vi "Main panel.vi"() -> ()   [LabVIEW 2019]
uses:
  <vilib>/Platform/TimedLoop/XDataNode/timing_clust.ctl
  <vilib>/Platform/TimedLoop/XDataNode/nitl_modes.ctl
  <vilib>/Platform/TimedLoop/XDataNode/wakeup.ctl
  <vilib>/myRIO/Instrument Drivers/Onboard IO/AI/typedefs/AI Reference.ctl
  <vilib>/myRIO/Common/Instrument Driver Framework/Utilities/typedefs/myRIO Generic Hardware Reference.ctl
  <vilib>/myRIO/Common/Instrument Driver Framework/Utilities/typedefs/Hardware Version Enum.ctl
  <vilib>/myRIO/Common/Instrument Driver Framework/Utilities/typedefs/myRIO v1.0 Reference.ctl
  <vilib>/myRIO/Common/Instrument Driver Framework/Utilities/typedefs/Generic FPGA Reference.ctl
  <vilib>/myRIO/Common/Instrument Driver Framework/myRIO v1.0/AI/typedefs/AI Channels List.ctl
  <vilib>/myRIO/Common/Instrument Driver Framework/myRIO v1.0/AI/typedefs/AI Channels Enum.ctl
  <vilib>/myRIO/Common/Instrument Driver Framework/Utilities/typedefs/Analog Scaling Constants List.ctl
  <vilib>/myRIO/Common/Instrument Driver Framework/Utilities/typedefs/Analog Scaling Constants.ctl
  <vilib>/userdefined/High Color/nirio_resource_hc.ctl
  <vilib>/myRIO/Instrument Drivers/Onboard IO/AO/typedefs/AO Reference.ctl
  <vilib>/myRIO/Common/Instrument Driver Framework/myRIO v1.0/AO/typedefs/AO Channels List.ctl
  <vilib>/myRIO/Common/Instrument Driver Framework/myRIO v1.0/AO/typedefs/AO Channels Enum.ctl
  <vilib>/myRIO/Common/Instrument Driver Framework/Utilities/vis/Is FPGA Ref Available.vi
  <vilib>/myRIO/Common/Instrument Driver Framework/myRIO v1.0/AI/vis/myRIO v1.1 Open AI.vi
  <vilib>/myRIO/Instrument Drivers/Onboard IO/AI/vis/Read.vi
  <vilib>/myRIO/Common/Instrument Driver Framework/myRIO v1.0/AO/vis/myRIO v1.1 Open AO.vi
  <vilib>/myRIO/Instrument Drivers/Onboard IO/AO/vis/Write.vi
  <vilib>/myRIO/Common/Instrument Driver Framework/Utilities/vis/Validate Channels.vi
  <vilib>/myRIO/Common/Instrument Driver Framework/myRIO v1.0/AI/vis/myRIO v1.0 Reserve AI.vi
  <vilib>/myRIO/Common/Instrument Driver Framework/myRIO v1.0/AO/vis/myRIO v1.0 Reserve AO.vi
  <vilib>/myRIO/Common/Instrument Driver Framework/myRIO v1.0/UART/vis/myRIO v1.0 Close UART.vi
  <vilib>/myRIO/Common/Instrument Driver Framework/myRIO v1.0/AI/vis/myRIO v1.0 Build MUX Configuration AI.vi
  <vilib>/myRIO/Common/Instrument Driver Framework/myRIO v1.0/Resource Manager/vis/myRIO v1.0 Reserve Channel List.vi
  <vilib>/myRIO/Common/Instrument Driver Framework/myRIO v1.0/AO/vis/myRIO v1.0 Build MUX Configuration AO.vi
  <vilib>/myRIO/Common/Instrument Driver Framework/myRIO v1.0/Resource Manager/vis/myRIO v1.0 Reserve Channel.vi
  <vilib>/myRIO/Common/Instrument Driver Framework/myRIO v1.0/Resource Manager/vis/myRIO v1.0 Unreserve Channel.vi
  <vilib>/myRIO/Common/Instrument Driver Framework/myRIO v1.0/Resource Manager/vis/myRIO v1.0 Build Mutex Name.vi
  Global.vi
  <vilib>/Utility/VariantDataType/GetNumericInfo.vi
  <vilib>/Utility/error.llb/Error Cluster From Error Code.vi
  <vilib>/myRIO/Common/Instrument Driver Framework/myRIO v1.0/myRIO v1.1 Open.vi
  <vilib>/myRIO/Common/Instrument Driver Framework/myRIO v1.0/AI/vis/myRIO v1.0 Get Scaling Constants AI.vi
  <vilib>/myRIO/Common/Instrument Driver Framework/Utilities/vis/IO Manager.vi
  <vilib>/myRIO/Common/Instrument Driver Framework/Utilities/vis/Configuration Manager.vi
  <vilib>/myRIO/Common/Instrument Driver Framework/myRIO v1.0/myRIO v1.0 Close.vi
  <vilib>/myRIO/Common/Instrument Driver Framework/myRIO v1.0/AI/vis/myRIO v1.0 Read AI.vi
  <vilib>/myRIO/Common/Instrument Driver Framework/myRIO v1.0/AO/vis/myRIO v1.0 Get Scaling Constants AO.vi
  <vilib>/myRIO/Common/Instrument Driver Framework/myRIO v1.0/AO/vis/myRIO v1.0 Write AO.vi
  <vilib>/myRIO/Common/Instrument Driver Framework/Utilities/vis/FPGA Ref Manager.vi
  <vilib>/myRIO/Common/Instrument Driver Framework/myRIO v1.0/myRIO v1.0 Reset FPGA.vi
  <vilib>/myRIO/Common/Instrument Driver Framework/myRIO v1.0/IRQ/vis/myRIO v1.0 IRQ Info FGV.vi
  <vilib>/myRIO/Common/Instrument Driver Framework/myRIO v1.0/IRQ/vis/myRIO v1.0 Timer IRQ Info FGV.vi
  <vilib>/myRIO/Common/Instrument Driver Framework/myRIO v1.0/IRQ/vis/myRIO v1.0 ISR Agent.vi
  <vilib>/myRIO/Instrument Drivers/Utilities/vis/Reset Index.vi
  <vilib>/myRIO/Common/Instrument Driver Framework/myRIO v1.0/Resource Manager/vis/myRIO v1.0 Block Write Resource Manager.vi
  <vilib>/platform/TimedLoop/XDataNode/XDataNode.xnode
  <vilib>/myRIO/Express VI/Onboard IO/AI/AI Express VI.xnode
  <vilib>/myRIO/Instrument Drivers/Onboard IO/AI/vis/myRIO AI Open.xnode
  <vilib>/myRIO/Express VI/Onboard IO/AO/AO Express VI.xnode
  <vilib>/myRIO/Instrument Drivers/Onboard IO/AO/vis/myRIO AO Open.xnode
  <vilib>/myRIO/Instrument Drivers/Utilities/Utilities.lvlib
  <vilib>/Platform/TimedLoop/XDataNode/XDNodeRunTimeDep.lvlib
  <vilib>/myRIO/Instrument Drivers/Onboard IO/AI/AI.lvlib
  <vilib>/myRIO/Instrument Drivers/Onboard IO/AO/AO.lvlib
  <vilib>/measure/NI_MABase.lvlib
panel:
  out "Data Collection":T1(graph)
  in  "Start":bool
  out "x/y":dbl
  out "Controller o/p":dbl
  in  "Sin wave":T2={"Frequency (Hz)"=3.3333e-05, "Amplitude"=0.14999999999999997, "Phase"=0.0, "offset"=0.6} {"offset" format="%0.2p"}
  in  "output range":cluster{"output high":dbl, "output low":dbl}={"output high"=200.0, "output low"=-100.0} {"output low" format="%.2f"; "output high" format="%.2f"}
  in  "PID gains":T3={"proportional gain (Kc)"=3.0, "integral time (Ti, min)"=0.01, "derivative time (Td, min)"=0.0} {"derivative time (Td, min)" format="%.6f"; "integral time (Ti, min)" format="%.6f"; "proportional gain (Kc)" format="%.3f"}
  out "Regulator Raw o/p":dbl
  in  "off/on":bool
  in  "Square wave":T4={"Frequency (Hz)"=1.2, "Delay"=30.0, "Duty cycle %"=55.0}
  out "Solenoid Signals":cluster{i16, i16}(graph)
  in  "manual P Value (bar)":dbl=0.71
  in  "PID/Auto":bool
  out "output y(t)":dbl
  in  "Tab Control":T5(tab)
  out "Pressure regulator signal":cluster{"f":dbl, "Angle rad":dbl, dbl, dbl}(graph)
  out "Pressure (Bar)":cluster{"outy":dbl, dbl, dbl}(graph)
  out "Pressure (Bar)":dbl
  in  "Regulator off/on":bool
  out "Time":dbl format="%<%H:%M:%S>t"
  in  "Period [s]":dbl=0.001
  in  "Stop Button":bool
  # "Square wave"
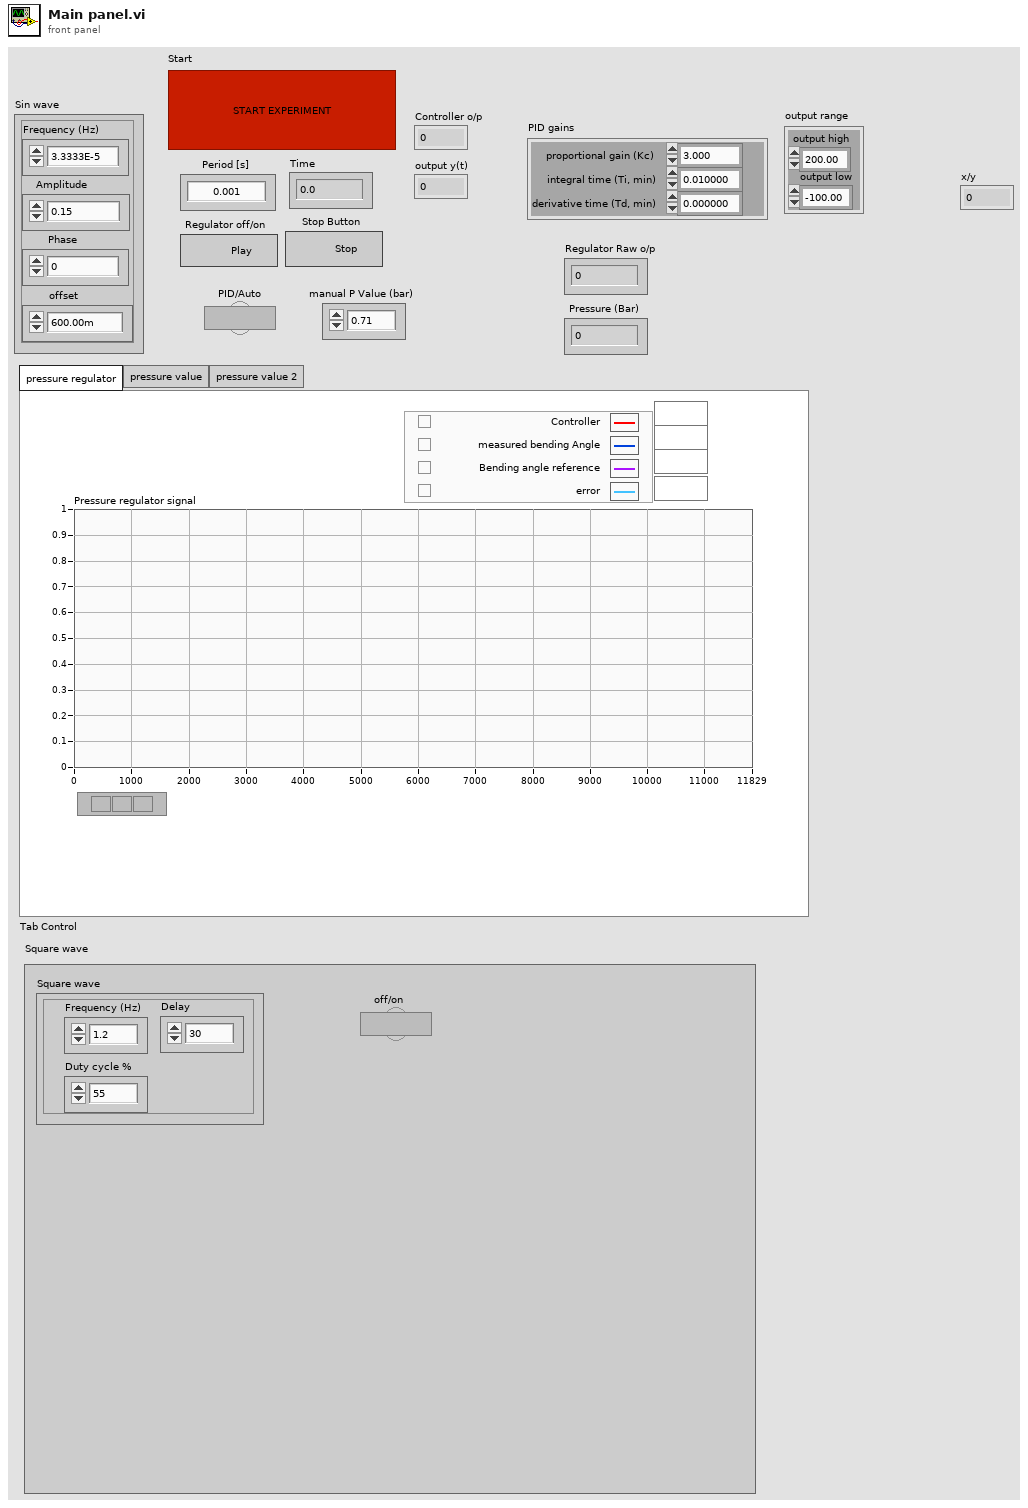
[diagram p1: front panel]
types:
  T1 = cluster{"B/AI0 (Pin 3)":dbl, "f":dbl, dbl, "Left":dbl, "Right":dbl, "Left":dbl, "Right":dbl, "L&R":dbl, "Envelope":dbl, dbl, dbl}
  T2 = cluster{"Frequency (Hz)":dbl, "Amplitude":dbl, "Phase":dbl, "offset":dbl}
  T3 = cluster{"proportional gain (Kc)":dbl, "integral time (Ti, min)":dbl, "derivative time (Td, min)":dbl}
  T4 = cluster{"Frequency (Hz)":dbl, "Delay":dbl, "Duty cycle %":dbl}
  T5 = enum32{"pressure regulator", "pressure value", "pressure value 2"}
  T6 = cluster{"B/AI0 (Pin 3)":dbl, "f":dbl, dbl, "Left":dbl, "Right":dbl, "Left":dbl, "Right":dbl, "L&R":dbl, "Envelope":dbl, dbl, dbl}[]
  T7 = cluster{"dbl Scaled Value":dbl, "dbl Scaled Value":dbl}[]
  T8 = typedef "AO.lvlib/AO Reference.ctl" = cluster{"myRIO Reference":T9, "AO Channel List":T13, "AO Scaling Constant List":T15}
  T9 = typedef "myRIO Generic Hardware Reference.ctl" = cluster{"myRIO Model":T10, "myRIO Hardware Reference":T11}
  T10 = typedef "Hardware Version Enum.ctl" = enum16{"Unknown", "myRIO-1900", "myRIO-1950", "roboRIO", "NI ELVIS RIO CM", "ELVIS III"}
  T11 = typedef "myRIO v1.0 Reference.ctl" = cluster{"Generic FPGA Reference":T12, "Allow multiple opens":bool}
  T12 = typedef "Generic FPGA Reference.ctl" = refnum<k20>
  T13 = typedef "AO Channels List.ctl" = T14[]
  T14 = typedef "AO Channels Enum.ctl" = enum16{"Not Connected", "AudioOut/Left", "AudioOut/Right", "C/AO0", "C/AO1", "A/AO0", "A/AO1", "B/AO0", "B/AO1"}
  T15 = typedef "Analog Scaling Constants List.ctl" = T16[]
  T16 = typedef "Analog Scaling Constants.ctl" = cluster{"LSB Weight (Volts)":dbl, "Offset (Volts)":dbl, "Signed?":bool}
  T17 = typedef "nirio_resource_hc.ctl" = tag
  T18 = typedef "AI.lvlib/AI Reference.ctl" = cluster{"myRIO Reference":T9, "AI Channels List":T19, "AI Scaling Constants List":T15}
  T19 = typedef "AI Channels List.ctl" = T20[]
  T20 = typedef "AI Channels Enum.ctl" = enum16{"Not Connected", "AudioIn/Left", "AudioIn/Right", "C/AI0", "C/AI1", "A/AI0", "A/AI1", "A/AI2", "A/AI3", "A/AI4", "A/AI5", "A/AI6", "A/AI7", "B/AI0", "B/AI1", "B/AI2", "B/AI3", "B/AI4", "B/AI5", "B/AI6", "B/AI7", "AI/AI0", "AI/AI1", "AI/AI2", "AI/AI3", "A/AI0 (DIFF)", "A/AI1 (DIFF)", "A/AI2 (DIFF)", "A/AI3 (DIFF)", "B/AI0 (DIFF)", "B/AI1 (DIFF)", "B/AI2 (DIFF)", "B/AI3 (DIFF)"}
  T21 = typedef "XDNodeRunTimeDep.lvlib/timing_clust.ctl" = cluster{"Expected End [f-1]":u64, "Actual End [f-1]":u64, "Finished Late? [f-1]":bool, "Expected End [i-1]":u64, "Actual End [i-1]":u64, "Finished Late? [i-1]":bool, "Expected Start [i]":u64, "Actual Start [i]":u64, "Expected Start [f]":u64, "Actual Start [f]":u64, "Source Name":string, "Structure Name":string, "Period":i64, "Deadline":i64, "Offset":i64, "Start":i64, "Priority":i32, "Timeout":i32, "Mode":T22, "Wakeup Reason":T23, "Error":errorcluster, "Source Type":string, "Secondary Source Type":string, "Global End Time":u64, "Global Start Time":u64, "Frame Duration":u64, "Iteration Duration":u64, "Assigned CPU":i32, "I/O Scan Engine Mode":u32}
  T22 = typedef "XDNodeRunTimeDep.lvlib/nitl_modes.ctl" = enum32{"No Change", "Process missed periods, maintain original phase", "Discard missed periods, maintain original phase", "Process missed periods, ignore original phase", "Discard missed periods, ignore original phase"}
  T23 = typedef "XDNodeRunTimeDep.lvlib/wakeup.ctl" = enum32{"Normal", "Aborted", "Asynchronous wakeup", "Timing source error", "Timed loop error", "Timeout"}
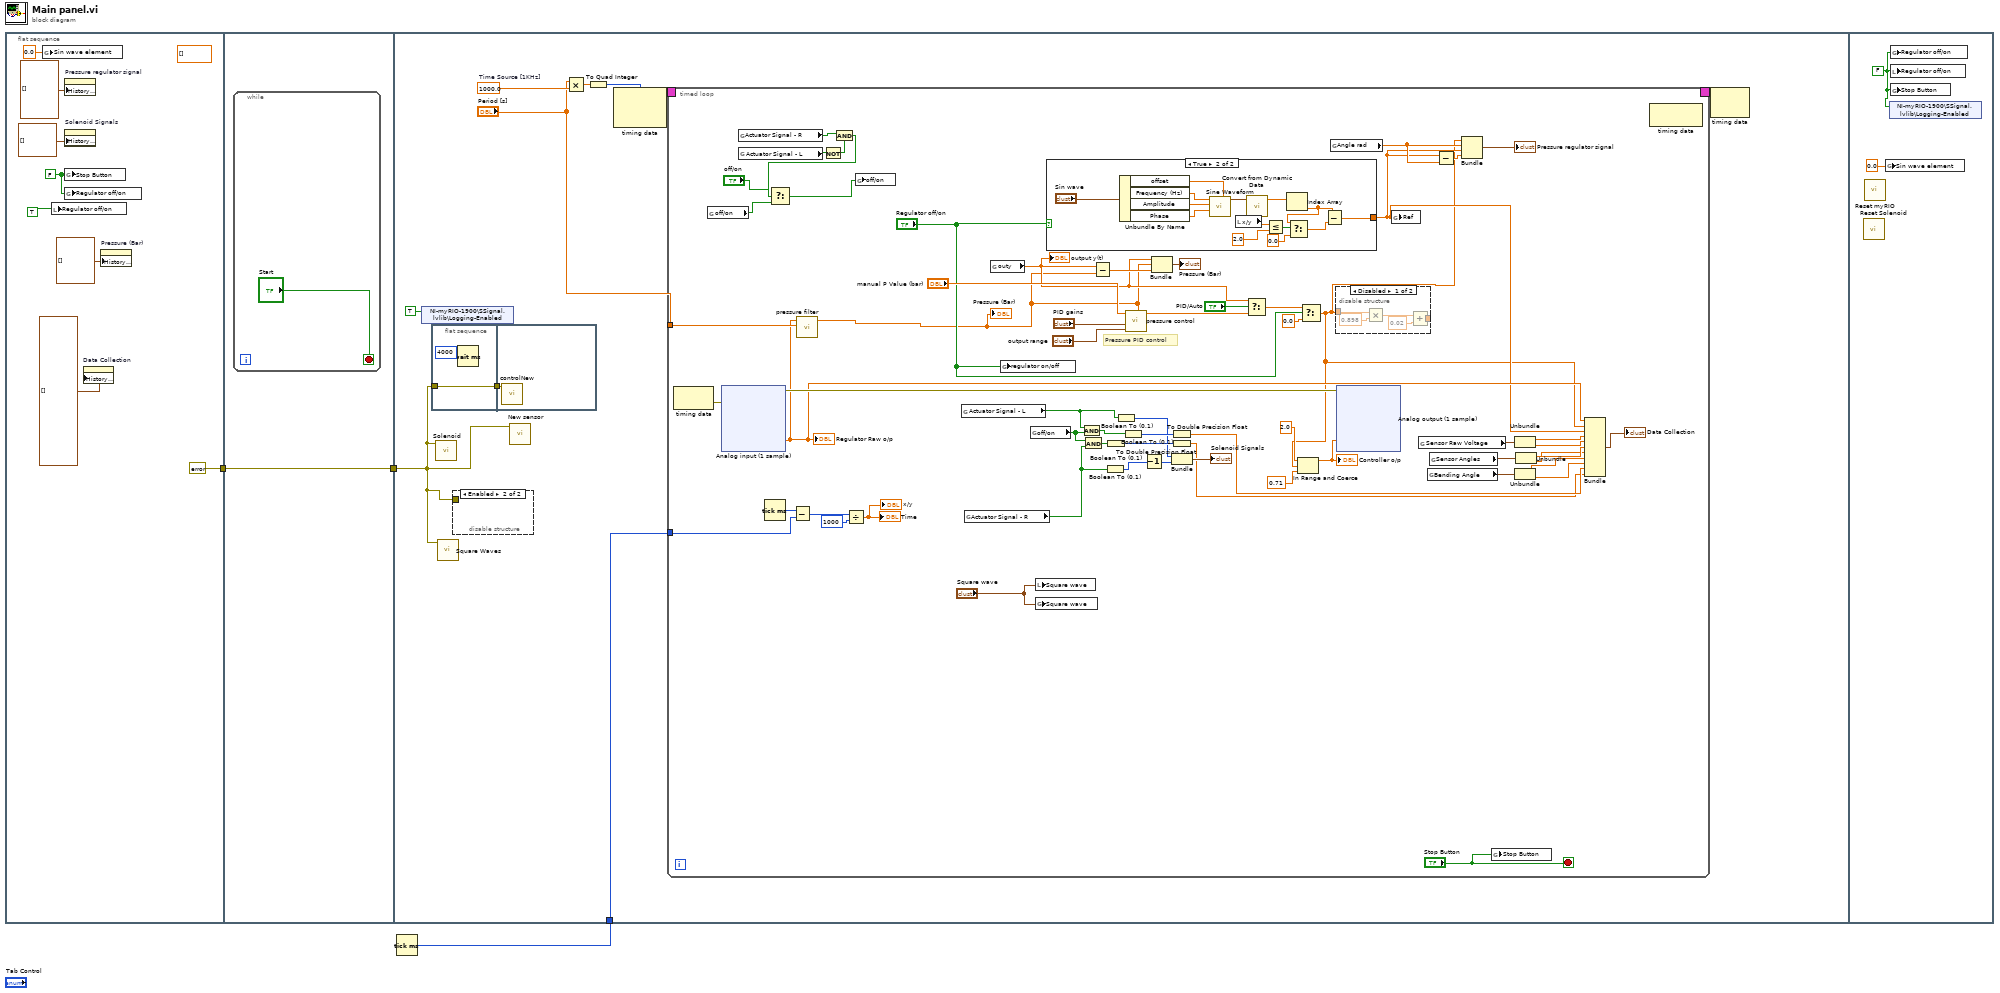
[diagram p0: block diagram]
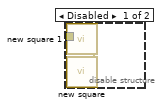
[diagram p2: hidden frame]
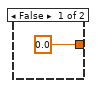
[diagram p4: hidden frame]
diagram:
  n1 = flat-sequence {
    tunnel: [errorcluster {"status"=FALSE, "code"=0, "source"=""} ("error constant")] -> w2
    tunnel: w2 -> [w12]
    tunnel: [w12] -> w1
    tunnel: w3 -> [w18]
    tunnel: w1 -> [w15]
    frame #0 {
      (unwired) dbl[] [] ("History Data")
      w10 = FALSE ("Stop Button")
      n2 = global write "Global.vi" "Sin wave element"(0.0 ("pressure regulator")) -> ()
      n3 = local write "Regulator off/on"(TRUE ("Regulator off/on")) -> ()
      n4 = property on="Pressure regulator signal" class="WFChart (strict)"("History Data"=cluster{"f":dbl, "Angle rad":dbl, dbl, dbl}[] []) -> ()  [unwired: 2 in, 2 out]
      n5 = property on="Solenoid Signals" class="WFChart (strict)"("History Data"=T7 []) -> ()  [unwired: 2 in, 2 out]
      n6 = global write "Global.vi" "Stop Button"(w10) -> ()
      n7 = global write "Global.vi" "Regulator off/on"(w10) -> ()
      n8 = property on="Data Collection" class="WFChart (strict)"("History Data"=T6 []) -> ()  [unwired: 2 in, 2 out]
      n9 = property on="Pressure (Bar)" class="WFChart (strict)"("History Data"=cluster{"outy":dbl, dbl, dbl}[] []) -> ()  [unwired: 2 in, 2 out]
    }
    frame #1 {
      n10 = while {
        stop <- "Start" stop-if-true
      }
    }
    frame #2 {
      w21 = 1000.0  # Time Source [1KHz]
      n11 = shared-variable "NI-myRIO-1900\\SSignal.lvlib\\Logging-Enabled"(TRUE ("Logging-Enabled")) -> ()  [unwired: 1 in, 1 out]
      n12 = flat-sequence {
        tunnel: w15 -> [w25]
        tunnel: [w25] -> w14
        tunnel: w14 -> [w26]
        frame #0 {
          n13 = Wait (ms)(milliseconds to wait=u32 4000) -> ()  [unwired: 1 out]
        }
        frame #1 {
          n14 = call "controlNew.vi"("Error In"=w26) -> ()  [unwired: 10 in, 1 out]
        }
      }
      n15 = call "Solenoid.vi"("Error In"=w15) -> ()  [unwired: 11 in]
      n16 = call "Square Waves.vi"("Error In"=w15) -> ()  [unwired: 11 in]
      n17 = disable-structure shown="Enabled" {
        disable-tunnel: w15 -> [w27 _]
        frame Disabled {
          n18 = call "new square 1.vi"("Error In"=w27) -> ()  [unwired: 11 in]
          n19 = call "new square.vi"("Error In"=w27) -> ()  [unwired: 11 in]
        }
        frame Enabled {
        }
      }
      n20 = call "New sensor.vi"("error in (no error)"=w15) -> ()  [unwired: 10 in, 1 out]
      n21 = Multiply(x="Period [s]", y=w21) -> (x*y=w20:dbl)
      n22 = To Quad Integer(1:w20) -> (0:w19:i64)
      n23 = node-c288(w19) -> (w23:T21)  [unwired: 1 in]
      n24 = timed-loop {
        timing: w23 -> [_]
        timing-out: [_] -> w22
        tunnel: w18 -> [w83]
        tunnel: "Period [s]" -> [w77]
        stop <- "Stop Button" stop-if-true
        # "Pressure PID control"
        n25 = node-c288() -> (w82:errorcluster)  [unwired: 1 in]
        n26 = global read "Global.vi" "off/on"() -> (w30:bool)
        n27 = xnode "Analog input (1 sample)"("error in (no error)"=w82) -> ("B/AI0 (Pin 3)"=w59:dbl, "error out"=w75:errorcluster)
        "Regulator Raw o/p" <- w59
        n28 = global read "Global.vi" "Actuator Signal - R"() -> (w33:bool)
        n29 = global read "Global.vi" "Actuator Signal - L"() -> (w35:bool)
        n30 = Tick Count (ms)() -> (millisecond timer value=w87:u32)
        n31 = Subtract(x=w87, y=w83) -> (x-y=w86:u32)
        n32 = call "pressure filter.vi"("Ts"=w77, "P"=w59) -> ("P"=w63:dbl)  [unwired: 9 in]
        "Pressure (Bar)" <- w63
        n33 = Not(x=w35) -> (.not. x?=w34:bool)
        n34 = And(x=w33, y=w34) -> (x .and. y?=w32:bool)
        n35 = Select(t="off/on", s=w32, f=w30) -> (s? t:f=w29:bool)
        n36 = Divide(x=w86, y=u32 1000) -> (x/y=→"Time" →"x/y":dbl)
        n37 = global write "Global.vi" "off/on"(w29) -> ()
        n38 = global read "Global.vi" "Actuator Signal - L"() -> (w36:bool)
        n39 = global read "Global.vi" "Actuator Signal - R"() -> (w38:bool)
        n40 = global read "Global.vi" "outy"() -> (w64:dbl)
        "output y(t)" <- w64
        n41 = global write "Global.vi" "regulator on/off"("Regulator off/on") -> ()
        n42 = global read "Global.vi" "off/on"() -> (w41:bool)
        n43 = local write "Square wave"("Square wave") -> ()
        n44 = global write "Global.vi" "Square wave"("Square wave") -> ()
        n45 = case shown="True" "Regulator off/on" {
          tunnel: [0.0 w99] -> w58
          frame False {
          }
          frame True {
            n46 = Unbundle By Name("Sin wave") -> ("offset"=w103:dbl, "Frequency (Hz)"=w106:dbl, "Amplitude"=w107:dbl, "Phase"=w105:dbl)
            n47 = call <vilib>:"Sine Waveform.vi"("offset"=w103, "phase"=w105, "amplitude"=w107, "frequency"=w106) -> ("signal out"=w108:waveform(dbl))  [unwired: 6 in, 1 out]
            n48 = local read "x/y"() -> (w101:dbl)
            n49 = call "Convert from Dynamic Data"("Dynamic Data Type"=w108) -> ("Array"=w95:dbl[])  [unwired: 3 in]
            n50 = Less Or Equal?(x=w101, y=2.0) -> (x <= y?=w102:bool)
            n51 = Index Array(array=w95) -> (element=w96:dbl)  [unwired: 1 in]
            n52 = Select(t=w96, s=w102, f=0.0) -> (s? t:f=w98:dbl)
            n53 = Subtract(x=w96, y=w98) -> (x-y=w99:dbl)
          }
        }
        n54 = And(x=w36, y=w41) -> (x .and. y?=w43:bool)
        n55 = And(x=w41, y=w38) -> (x .and. y?=w42:bool)
        n56 = Subtract(x=w64, y=w63) -> (x-y=w69:dbl)
        n57 = Boolean To (0,1)(Boolean=w38) -> (0, 1=w39:i16)
        n58 = Boolean To (0,1)(Boolean=w42) -> (0, 1=w40:i16)
        n59 = Boolean To (0,1)(Boolean=w36) -> (0, 1=w37:i16)
        n60 = Boolean To (0,1)(Boolean=w43) -> (0, 1=w71:i16)
        n61 = call "pressure control.vi"("output range"="output range", "PID gains"="PID gains", "process variable"=w63, "setpoint"="manual P Value (bar)") -> ("output"=w78:dbl)  [unwired: 7 in]
        n62 = Decrement(x=w39) -> (x-1=w70:i16)
        n63 = Bundle("outy"=w64, "P"=w63, w69) -> (→"Pressure (Bar)":cluster{"outy":dbl, "P":dbl, dbl})  [unwired: 1 in]
        n64 = To Double Precision Float(number=w71) -> (double precision float=w46:dbl)
        n65 = To Double Precision Float(number=w40) -> (double precision float=w45:dbl)
        n66 = Bundle(w37, w70) -> (→"Solenoid Signals":cluster{i16, i16})  [unwired: 1 in]
        n67 = Select(t=w64, s="PID/Auto", f=w78) -> (s? t:f=w76:dbl)
        n68 = Select(t=w76, s="Regulator off/on", f=0.0) -> (s? t:f=w28:dbl)
        n69 = In Range and Coerce(upper limit=2.0, x=w28, lower limit=0.71) -> (coerced(x)=w57:dbl)  [unwired: 1 out]
        "Controller o/p" <- w57
        n70 = global read "Global.vi" "Angle rad"() -> (w67:dbl)
        n71 = disable-structure shown="Disabled" {
          disable-tunnel: [w90 _] -> _
          disable-tunnel: w28 -> [w89 _]
          frame Disabled {
            n72 = Multiply(x=w89, y=0.898) -> (x*y=w93:dbl)
            n73 = Add(x=w93, y=0.02) -> (x+y=w90:dbl)
          }
          frame Enabled {
          }
        }
        n74 = xnode "Analog output (1 sample)"("C/AO0 (AO0)"=w57, "error in (no error)"=w75) -> ()  [unwired: 1 out]
        n75 = global write "Global.vi" "Ref"(w58) -> ()
        n76 = global read "Global.vi" "Sensor Raw Voltage"() -> (w55:cluster{"Left":dbl, "Right":dbl})
        n77 = global read "Global.vi" "Bending Angle"() -> (w49:cluster{"L&R":dbl, "Envelope":dbl})
        n78 = global read "Global.vi" "Sensor Angles"() -> (w52:cluster{"Left":dbl, "Right":dbl})
        n79 = Subtract(x=w58, y=w67) -> (x-y=w68:dbl)
        n80 = Bundle("f"=w28, "Angle rad"=w67, w58, w68) -> (→"Pressure regulator signal":cluster{"f":dbl, "Angle rad":dbl, dbl, dbl})  [unwired: 1 in]
        n81 = global write "Global.vi" "Stop Button"("Stop Button") -> ()
        n82 = Unbundle(w55) -> ("Left"=w54:dbl, "Right"=w53:dbl)
        n83 = Unbundle(w49) -> ("L&R"=w48:dbl, "Envelope"=w47:dbl)
        n84 = Unbundle(w52) -> ("Left"=w51:dbl, "Right"=w50:dbl)
        n85 = Bundle("B/AI0 (Pin 3)"=w59, "f"=w28, w58, "Left"=w54, "Right"=w53, "Left"=w51, "Right"=w50, "L&R"=w48, "Envelope"=w47, w46, w45) -> (→"Data Collection":T1)  [unwired: 1 in]
        n86 = node-c288() -> ()  [unwired: 1 in, 1 out]
      }
      n87 = node-c288(w22) -> ()  [unwired: 1 out]
    }
    frame #3 {
      w190 = FALSE ("Regulator off/on")
      n88 = call "Reset Solenoid.vi"() -> ()  [unwired: 12 in]
      n89 = call <vilib>:"Reset myRIO.vi"() -> ()  [unwired: 11 in, 1 out]
      n90 = global write "Global.vi" "Sin wave element"(0.0 ("pressure regulator")) -> ()
      n91 = shared-variable "NI-myRIO-1900\\SSignal.lvlib\\Logging-Enabled"(w190) -> ()  [unwired: 1 in, 1 out]
      n92 = global write "Global.vi" "Regulator off/on"(w190) -> ()
      n93 = local write "Regulator off/on"(w190) -> ()
      n94 = global write "Global.vi" "Stop Button"(w190) -> ()
    }
  }
  n95 = Tick Count (ms)() -> (millisecond timer value=w3:u32)
